vi "roboRIO v1.0 Build MUX Configuration DIO.vi"(11 "DIO Channel List":T4) -> (2 "Configuration Bitmask Array":bool[][](array[boolean]), 3 "Channel Reservation List":T1)   [LabVIEW 2021]
uses:
  <vilib>/myRIO/Common/Instrument Driver Framework/myRIO v1.0/DIO/typedefs/DIO Channels List.ctl
  <vilib>/myRIO/Common/Instrument Driver Framework/myRIO v1.0/DIO/typedefs/DIO Channels Enum.ctl
  <vilib>/myRIO/Common/Instrument Driver Framework/roboRIO v1.0/Resource Manager/typedefs/roboRIO v1.0 Channel Reservation List.ctl
  <vilib>/myRIO/Common/Instrument Driver Framework/roboRIO v1.0/Resource Manager/typedefs/roboRIO v1.0 Channel Reservation Info.ctl
  <vilib>/myRIO/Common/Instrument Driver Framework/roboRIO v1.0/Resource Manager/typedefs/roboRIO v1.0 Connector List.ctl
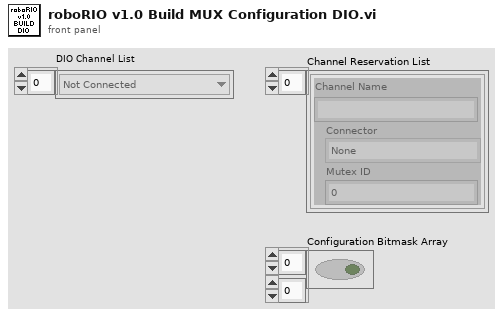
[diagram p1: front panel]
types:
  T1 = typedef "roboRIO v1.0 Channel Reservation List.ctl" = T2[]
  T2 = typedef "roboRIO v1.0 Channel Reservation Info.ctl" = cluster{"Channel Name":string, "Connector":T3, "Mutex ID":i32}
  T3 = typedef "roboRIO v1.0 Connector List.ctl" = enum32{"None", "ConnectorB", "ConnectorI2C", "ConnectorDIO", "ConnectorRSL", "ConnectorRELAY", "ConnectorAI", "ConnectorPWM", "ConnectorSPI"}
  T4 = typedef "DIO Channels List.ctl" = T5[]
  T5 = typedef "DIO Channels Enum.ctl" = enum16{"Not Connected", "C/DIO0", "C/DIO1", "C/DIO2", "C/DIO3", "C/DIO4", "C/DIO5", "C/DIO6", "C/DIO7", "A/DIO0", "A/DIO1", "A/DIO2", "A/DIO3", "A/DIO4", "A/DIO5", "A/DIO6", "A/DIO7", "A/DIO8", "A/DIO9", "A/DIO10", "A/DIO11", "A/DIO12", "A/DIO13", "A/DIO14", "A/DIO15", "A/DIO16", "A/DIO17", "A/DIO18", "A/DIO19", "B/DIO0", "B/DIO1", "B/DIO2", "B/DIO3", "B/DIO4", "B/DIO5", "B/DIO6", "B/DIO7", "B/DIO8", "B/DIO9", "B/DIO10", "B/DIO11", "B/DIO12", "B/DIO13", "B/DIO14", "B/DIO15", "B/DIO16", "B/DIO17", "B/DIO18", "B/DIO19", "LED0", "LED1", "LED2", "LED3", "Button0", "DIO/DIO0", "DIO/DIO1", "DIO/DIO2", "DIO/DIO3", "DIO/DIO4", "DIO/DIO5", "DIO/DIO6", "DIO/DIO7", "DIO/DIO8", "DIO/DIO9", "SPI/CS0", "SPI/CS1", "SPI/CS2", "SPI/CS3", "LED RADIO (Green)", "LED RADIO (Red)", "LED COMM (Green)", "LED COMM (Red)", "LED MODE (Green)", "LED MODE (Red)"}
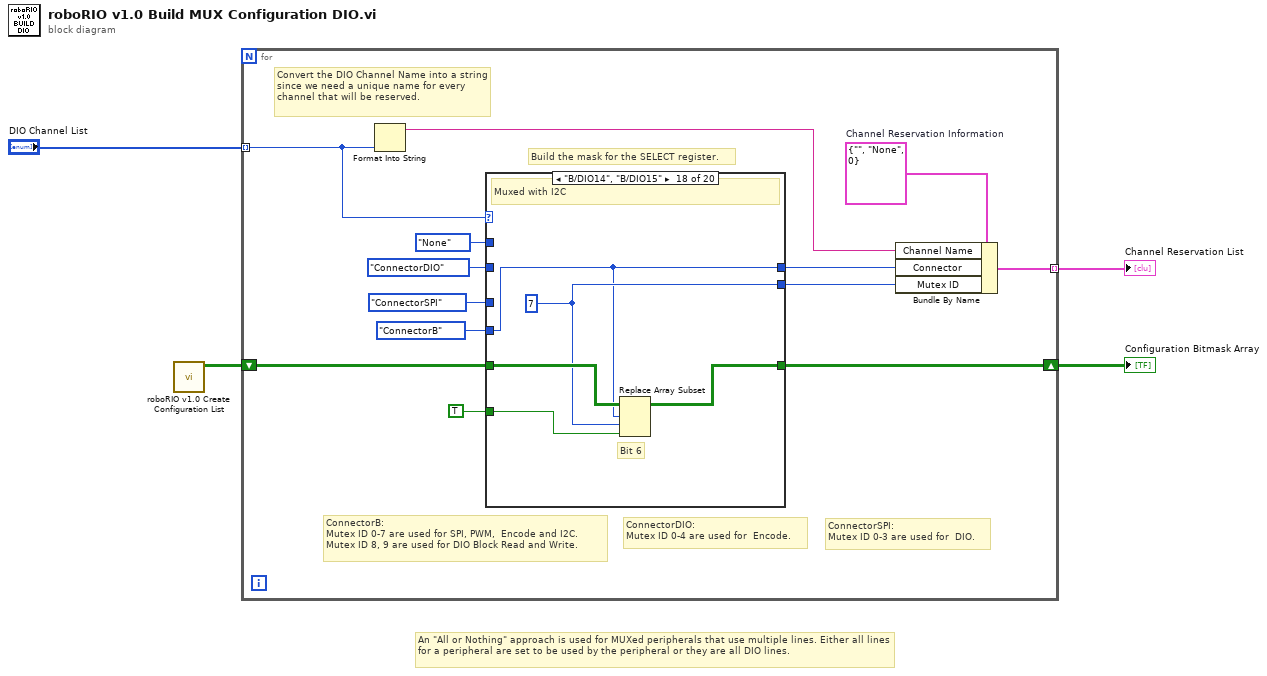
[diagram p0: block diagram]
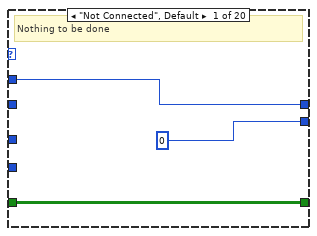
[diagram p2: hidden frame]
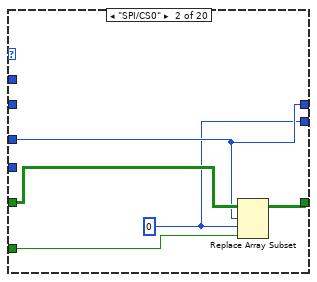
[diagram p3: hidden frame]
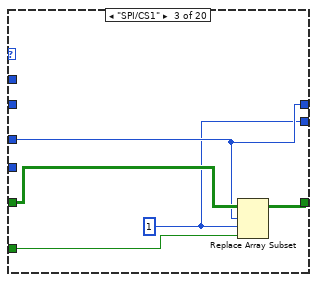
[diagram p4: hidden frame]
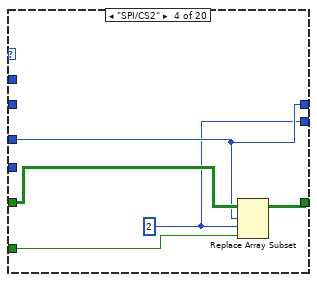
[diagram p5: hidden frame]
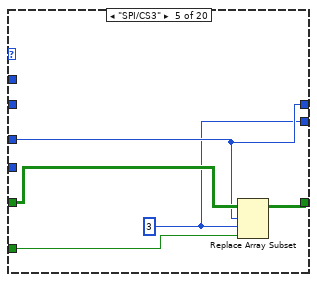
[diagram p6: hidden frame]
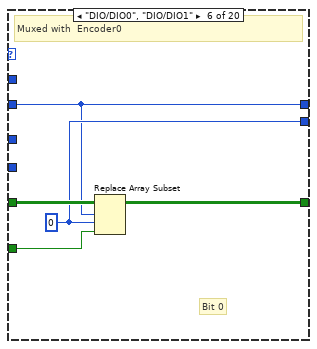
[diagram p7: hidden frame]
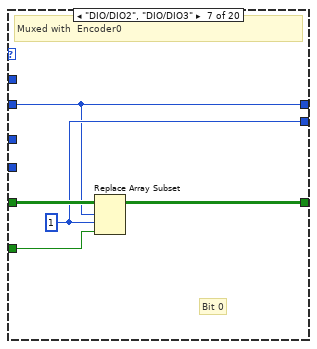
[diagram p8: hidden frame]
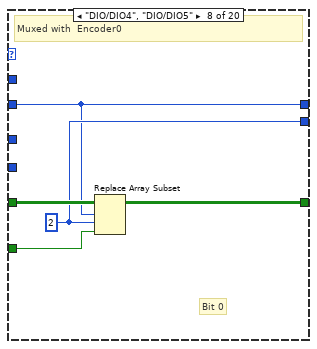
[diagram p9: hidden frame]
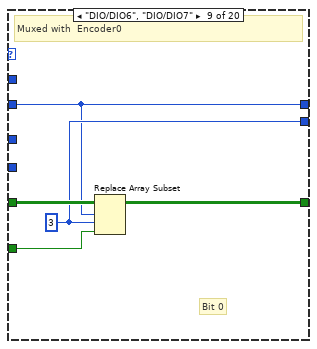
[diagram p10: hidden frame]
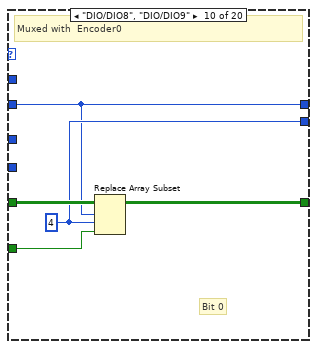
[diagram p11: hidden frame]
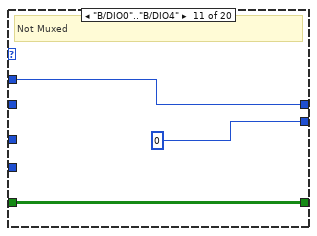
[diagram p12: hidden frame]
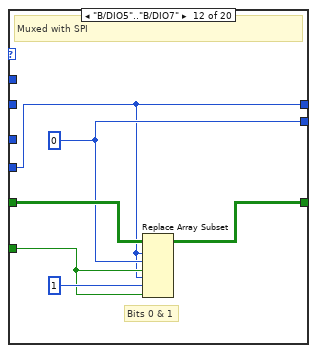
[diagram p13: hidden frame]
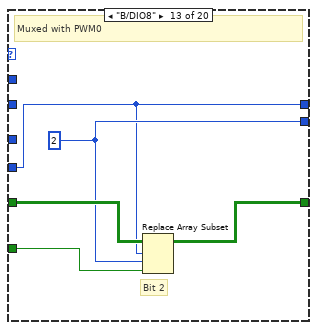
[diagram p14: hidden frame]
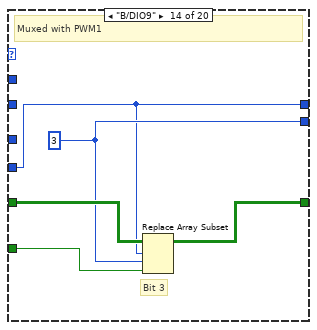
[diagram p15: hidden frame]
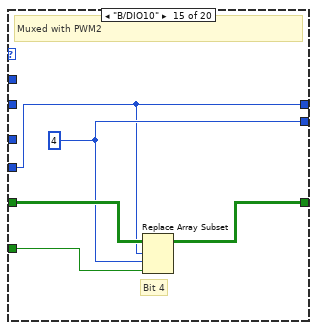
[diagram p16: hidden frame]
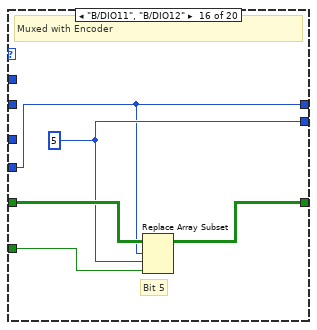
[diagram p17: hidden frame]
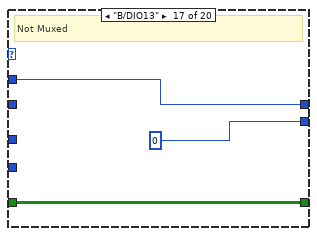
[diagram p18: hidden frame]
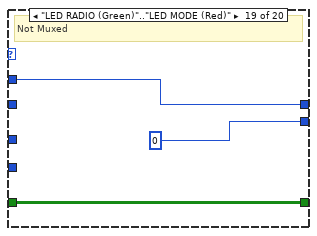
[diagram p19: hidden frame]
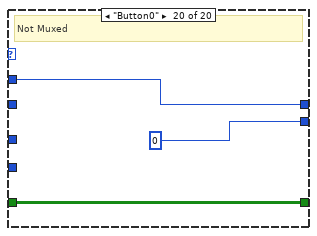
[diagram p20: hidden frame]
diagram:
  # "An \"All or Nothing\" approach is used for MUXed peripherals that use multiple lines. Either all lines for a peripheral are set to be used by the peripheral or they are all DIO lines."
  n1 = call <vilib>:"roboRIO v1.0 Create Configuration List.vi"() -> ("Bitmask Array"=w4:bool[][])  [unwired: 11 in]
  n2 = for {
    shift-right: [w14] -> w3
    shift-left: w4 -> [w15]
    tunnel: "DIO Channel List" -> [w9] mode=indexing
    tunnel: [w10] -> w1 mode=indexing
    w13 = T2 {"Channel Name"="", "Connector"=enum."None", "Mutex ID"=0}  # Channel Reservation Information
    # "ConnectorSPI:\nMutex ID 0-3 are used for  DIO."
    # "ConnectorDIO:\nMutex ID 0-4 are used for  Encode."
    # "ConnectorB:\nMutex ID 0-7 are used for SPI, PWM,  Encode and I2C.\nMutex ID 8, 9 are used for DIO Block Read and Write."
    # "Convert the DIO Channel Name into a string since we need a unique name for every channel that will be reserved."
    # "Build the mask for the SELECT register."
    n3 = Format Into String(w9) -> (resulting string=w8:string)  [unwired: 3 in, 1 out]
    n4 = case shown="\"B/DIO14\", \"B/DIO15\"" w9 {
      tunnel: w15 -> [w20 w25 w30 w35 w40 w45 w50 w55 w60 w65 w68 w74 w79 w84 w89 w94 w97 w102 w105 w108]
      tunnel: [w20 w22 w27 w32 w37 w44 w49 w54 w59 w64 w68 w73 w78 w83 w88 w93 w97 w101 w105 w108] -> w14
      tunnel: roboRIO_v1.0_Connector_List."None" ("Connector List") -> [w19 _ _ _ _ _ _ _ _ _ w67 _ _ _ _ _ w95 _ w103 w106]
      tunnel: TRUE ("new element/subarray") -> [_ w23 w28 w33 w38 w41 w46 w51 w56 w61 _ w70 w76 w81 w86 w90 _ w98 _ _]
      tunnel: [0 ("index") w21 w26 w31 w36 w43 w48 w53 w58 w63 0 ("index") w71 w77 w82 w87 w92 0 ("index") w100 0 ("index") 0 ("index")] -> w11
      tunnel: [w19 w24 w29 w34 w39 w42 w47 w52 w57 w62 w67 w69 w75 w80 w85 w91 w95 w99 w103 w106] -> w12
      tunnel: roboRIO_v1.0_Connector_List."ConnectorDIO" ("Connector List") -> [_ _ _ _ _ w42 w47 w52 w57 w62 _ _ _ _ _ _ _ _ _ _]
      tunnel: roboRIO_v1.0_Connector_List."ConnectorB" ("Connector List") -> [_ _ _ _ _ _ _ _ _ _ _ w69 w75 w80 w85 w91 _ w99 _ _]
      tunnel: roboRIO_v1.0_Connector_List."ConnectorSPI" ("Connector List") -> [_ w24 w29 w34 w39 _ _ _ _ _ _ _ _ _ _ _ _ _ _ _]
      frame "Not Connected", Default {
        # "Nothing to be done"
      }
      frame "SPI/CS0" {
        w21 = 0 ("index")
        n5 = Replace Array Subset(array=w25, new element=w23, index (row)=w24, index (col)=w21) -> (w22:bool[][])
      }
      frame "SPI/CS1" {
        w26 = 1 ("index")
        n6 = Replace Array Subset(array=w30, new element=w28, index (row)=w29, index (col)=w26) -> (w27:bool[][])
      }
      frame "SPI/CS2" {
        w31 = 2 ("index")
        n7 = Replace Array Subset(array=w35, new element=w33, index (row)=w34, index (col)=w31) -> (w32:bool[][])
      }
      frame "SPI/CS3" {
        w36 = 3 ("index")
        n8 = Replace Array Subset(array=w40, new element=w38, index (row)=w39, index (col)=w36) -> (w37:bool[][])
      }
      frame "DIO/DIO0", "DIO/DIO1" {
        w43 = 0 ("index")
        # "Bit 0"
        # "Muxed with  Encoder0"
        n9 = Replace Array Subset(array=w45, new element=w41, index (row)=w42, index (col)=w43) -> (w44:bool[][])
      }
      frame "DIO/DIO2", "DIO/DIO3" {
        w48 = 1 ("index")
        # "Bit 0"
        # "Muxed with  Encoder0"
        n10 = Replace Array Subset(array=w50, new element=w46, index (row)=w47, index (col)=w48) -> (w49:bool[][])
      }
      frame "DIO/DIO4", "DIO/DIO5" {
        w53 = 2 ("index")
        # "Bit 0"
        # "Muxed with  Encoder0"
        n11 = Replace Array Subset(array=w55, new element=w51, index (row)=w52, index (col)=w53) -> (w54:bool[][])
      }
      frame "DIO/DIO6", "DIO/DIO7" {
        w58 = 3 ("index")
        # "Bit 0"
        # "Muxed with  Encoder0"
        n12 = Replace Array Subset(array=w60, new element=w56, index (row)=w57, index (col)=w58) -> (w59:bool[][])
      }
      frame "DIO/DIO8", "DIO/DIO9" {
        w63 = 4 ("index")
        # "Bit 0"
        # "Muxed with  Encoder0"
        n13 = Replace Array Subset(array=w65, new element=w61, index (row)=w62, index (col)=w63) -> (w64:bool[][])
      }
      frame "B/DIO0".."B/DIO4" {
        # "Not Muxed"
      }
      frame "B/DIO5".."B/DIO7" {
        w71 = 0 ("index")
        # "Bits 0 & 1"
        # "Muxed with SPI"
        n14 = Replace Array Subset(array=w74, new element #1=w70, index (row) #1=w69, index (col) #1=w71, new element #2=w70, index (row) #2=w69, index (col) #2=1 ("disabled index (col)")) -> (w73:bool[][])
      }
      frame "B/DIO8" {
        w77 = 2 ("index")
        # "Bit 2"
        # "Muxed with PWM0"
        n15 = Replace Array Subset(array=w79, new element=w76, index (row)=w75, index (col)=w77) -> (w78:bool[][])
      }
      frame "B/DIO9" {
        w82 = 3 ("index")
        # "Bit 3"
        # "Muxed with PWM1"
        n16 = Replace Array Subset(array=w84, new element=w81, index (row)=w80, index (col)=w82) -> (w83:bool[][])
      }
      frame "B/DIO10" {
        w87 = 4 ("index")
        # "Bit 4"
        # "Muxed with PWM2"
        n17 = Replace Array Subset(array=w89, new element=w86, index (row)=w85, index (col)=w87) -> (w88:bool[][])
      }
      frame "B/DIO11", "B/DIO12" {
        w92 = 5 ("index")
        # "Bit 5"
        # "Muxed with Encoder"
        n18 = Replace Array Subset(array=w94, new element=w90, index (row)=w91, index (col)=w92) -> (w93:bool[][])
      }
      frame "B/DIO13" {
        # "Not Muxed"
      }
      frame "B/DIO14", "B/DIO15" {
        w100 = 7 ("index")
        # "Bit 6"
        # "Muxed with I2C"
        n19 = Replace Array Subset(array=w102, new element=w98, index (row)=w99, index (col)=w100) -> (w101:bool[][])
      }
      frame "LED RADIO (Green)".."LED MODE (Red)" {
        # "Not Muxed"
      }
      frame "Button0" {
        # "Not Muxed"
      }
    }
    n20 = Bundle By Name(cluster=w13, "Channel Name"=w8, "Connector"=w12, "Mutex ID"=w11) -> (w10:T2)
  }
  "Configuration Bitmask Array" <- w3
  "Channel Reservation List" <- w1
